vi "Serialize as VTT.vi"(8 "error in (no error)":errorcluster, 11 "Element Array in":refnum<class "Element Array.lvclass">) -> (0 "error out":errorcluster, 2 "VTT Fragment":string, 3 "Element Array out":refnum<class "Element Array.lvclass">)   [LabVIEW 2018, in "VILab.lvlib" / "Element Array.lvclass"]
uses:
  Element Array.lvclass
  Element Array.lvclass/Element Array.ctl
  Attribute.lvclass
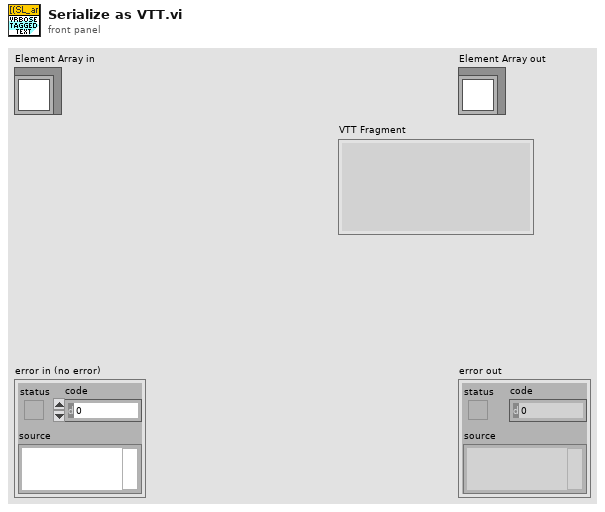
[diagram p1: front panel]
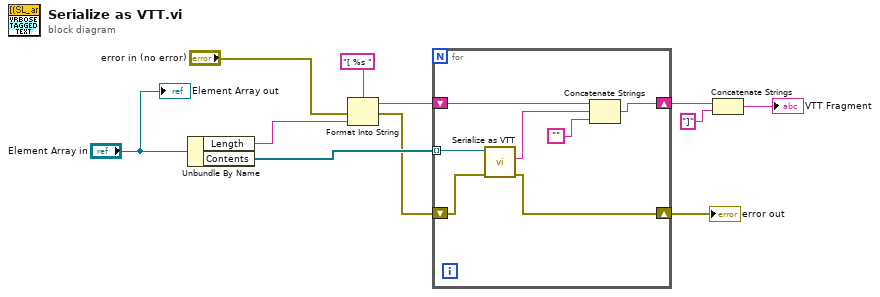
[diagram p0: block diagram]
diagram:
  n1 = Unbundle By Name("Element Array in") -> ("Length"=w1:string, "Contents"=w8:refnum<class "Attribute.lvclass">[])
  n2 = Format Into String(format string="[ %s ", error in="error in (no error)", w1) -> (resulting string=w7:string, error out=w6:errorcluster)  [unwired: 1 in]
  n3 = for {
    tunnel: w8 -> [w17] mode=indexing
    shift-right: [w13] -> w3
    shift-left: w7 -> [w18]
    shift-right: [w12] -> w5
    shift-left: w6 -> [w16]
    n4 = call-dynamic "Serialize as VTT.vi"("error in (no error)"=w16, "Attribute in"=w17) -> ("error out"=w12:errorcluster, "VTT Fragment"=w15:string)  [unwired: 7 in, 1 out]
    n5 = Concatenate Strings(w18, w15, "") -> (w13:string)
  }
  "error out" <- w5
  n6 = Concatenate Strings(w3, "]") -> (→"VTT Fragment":string)
  "Element Array out" <- "Element Array in"
